vi "rs3 capture single.vi"(0 "queue in":u64, 5 "timeout":u32=5000, 11 "error in (no error)":errorcluster) -> (1 "Capture Error":string="No Error", 3 "RS Format":u16(ring)=6 items=["    RS2_FORMAT_ANY             , /**< When passed to enable stream, librealsense will try to provide best suited format */", "    RS2_FORMAT_Z16             , /**< 16-bit linear depth values. The depth is meters is equal to depth scale * pixel value. */", "    RS2_FORMAT_DISPARITY16     , /**< 16-bit linear disparity values. The depth in meters is equal to depth scale / pixel value. */", "    RS2_FORMAT_XYZ32F          , /**< 32-bit floating point 3D coordinates. */", "    RS2_FORMAT_YUYV            , /**< Standard YUV pixel format as described in https://en.wikipedia.org/wiki/YUV */", "    RS2_FORMAT_RGB8            , /**< 8-bit red, green and blue channels */", "    RS2_FORMAT_BGR8            , /**< 8-bit blue, green, and red channels -- suitable for OpenCV */", "    RS2_FORMAT_RGBA8           , /**< 8-bit red, green and blue channels + constant alpha channel equal to FF */", "    RS2_FORMAT_BGRA8           , /**< 8-bit blue, green, and red channels + constant alpha channel equal to FF */", "    RS2_FORMAT_Y8              , /**< 8-bit per-pixel grayscale image */", "    RS2_FORMAT_Y16             , /**< 16-bit per-pixel grayscale image */", "    RS2_FORMAT_RAW10           , /**< Four 10-bit luminance values encoded into a 5-byte macropixel */", "    RS2_FORMAT_RAW16           , /**< 16-bit raw image */", "    RS2_FORMAT_RAW8            , /**< 8-bit raw image */", "    RS2_FORMAT_UYVY            , /**< Similar to the standard YUYV pixel format, but packed in a different order */", "    RS2_FORMAT_MOTION_RAW      , /**< Raw data from the motion sensor */", "    RS2_FORMAT_MOTION_XYZ32F   , /**< Motion data packed as 3 32-bit float values, for X, Y, and Z axis */", "    RS2_FORMAT_GPIO_RAW        , /**< Raw data from the external sensors hooked to one of the GPIO's */", "    RS2_FORMAT_COUNT             /**< Number of enumeration values. Not a valid input: intended to be used in for-loops. */"], 4 "RS Stream":u16(ring) items=["    RS2_STREAM_ANY,", "    RS2_STREAM_DEPTH                            , /**< Native stream of depth data produced by RealSense device */", "    RS2_STREAM_COLOR                            , /**< Native stream of color data captured by RealSense device */", "    RS2_STREAM_INFRARED                         , /**< Native stream of infrared data captured by RealSense device */", "    RS2_STREAM_FISHEYE                          , /**< Native stream of fish-eye (wide) data captured from the dedicate motion camera */", "    RS2_STREAM_GYRO                             , /**< Native stream of gyroscope motion data produced by RealSense device */", "    RS2_STREAM_ACCEL                            , /**< Native stream of accelerometer motion data produced by RealSense device */", "    RS2_STREAM_GPIO                             , /**< Signals from external device connected through GPIO */", "    RS2_STREAM_COUNT"], 6 "frame out":u64, 8 "width":i32, 10 "Stream type":u16(ring) items=["Depth"=0, "Color (ext.)"=2, "Color (left) "=3, "IR Left"=5, "IR Right"=9, "IR Left (Y16)"=21, "IR Right (Y16)"=25], 12 "index":i32, 14 "height":i32, 15 "error out":errorcluster)   [LabVIEW 2017, in "libRealSense3.lvlib"]
doc: "This VI waits for and returns the FRAME handle of captured data. \nIt also queries the frame profile to identify the type of stream data it was. \nThis type is output into the \"Stream Type\":\n\n0 Depth\n3 Color left\n5 IR Left \n9 IR Right\n21 IR Left (Y16)\n25 IR RIght (Y16)"
uses:
  libRealSense3.lvlib
panel:
  # "RS3 Capture Single"
  # "0   Depth\n3   Color left\n5   IR Left \n9  IR Right\n21  IR Left (Y16)\n25  IR RIght (Y16)"
  # "(C) Intel Corp. 2017,  AGJ"
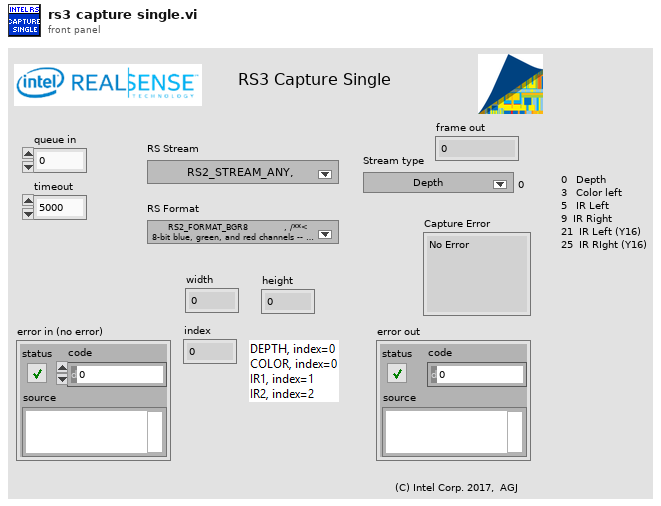
[diagram p1: front panel]
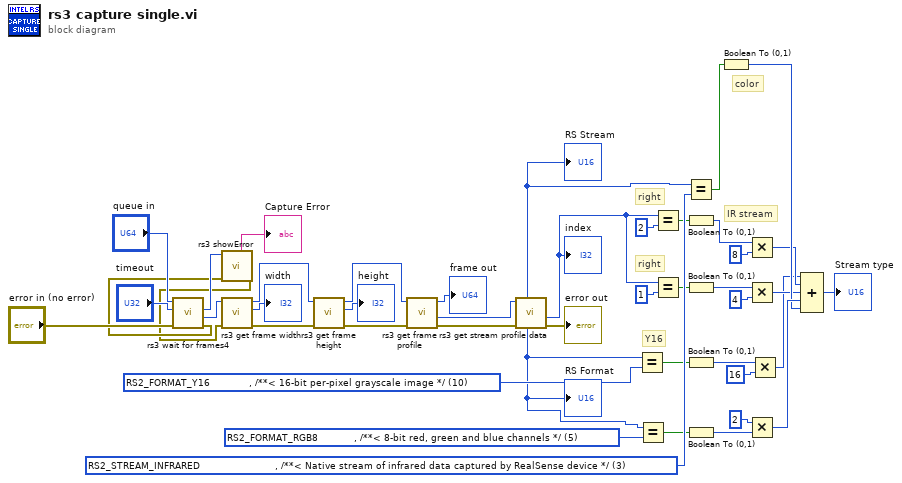
[diagram p0: block diagram]
diagram:
  w7 = u16 10 items=["    RS2_FORMAT_ANY             , /**< When passed to enable stream, librealsense will try to provide best suited format */", "    RS2_FORMAT_Z16             , /**< 16-bit linear depth values. The depth is meters is equal to depth scale * pixel value. */", "    RS2_FORMAT_DISPARITY16     , /**< 16-bit linear disparity values. The depth in meters is equal to depth scale / pixel value. */", "    RS2_FORMAT_XYZ32F          , /**< 32-bit floating point 3D coordinates. */", "    RS2_FORMAT_YUYV            , /**< Standard YUV pixel format as described in https://en.wikipedia.org/wiki/YUV */", "    RS2_FORMAT_RGB8            , /**< 8-bit red, green and blue channels */", "    RS2_FORMAT_BGR8            , /**< 8-bit blue, green, and red channels -- suitable for OpenCV */", "    RS2_FORMAT_RGBA8           , /**< 8-bit red, green and blue channels + constant alpha channel equal to FF */", "    RS2_FORMAT_BGRA8           , /**< 8-bit blue, green, and red channels + constant alpha channel equal to FF */", "    RS2_FORMAT_Y8              , /**< 8-bit per-pixel grayscale image */", "    RS2_FORMAT_Y16             , /**< 16-bit per-pixel grayscale image */", "    RS2_FORMAT_RAW10           , /**< Four 10-bit luminance values encoded into a 5-byte macropixel */", "    RS2_FORMAT_RAW16           , /**< 16-bit raw image */", "    RS2_FORMAT_RAW8            , /**< 8-bit raw image */", "    RS2_FORMAT_UYVY            , /**< Similar to the standard YUYV pixel format, but packed in a different order */", "    RS2_FORMAT_MOTION_RAW      , /**< Raw data from the motion sensor */", "    RS2_FORMAT_MOTION_XYZ32F   , /**< Motion data packed as 3 32-bit float values, for X, Y, and Z axis */", "    RS2_FORMAT_GPIO_RAW        , /**< Raw data from the external sensors hooked to one of the GPIO's */", "    RS2_FORMAT_COUNT             /**< Number of enumeration values. Not a valid input: intended to be used in for-loops. */"] ("RS Format")
  w29 = u16 3 items=["    RS2_STREAM_ANY,", "    RS2_STREAM_DEPTH                            , /**< Native stream of depth data produced by RealSense device */", "    RS2_STREAM_COLOR                            , /**< Native stream of color data captured by RealSense device */", "    RS2_STREAM_INFRARED                         , /**< Native stream of infrared data captured by RealSense device */", "    RS2_STREAM_FISHEYE                          , /**< Native stream of fish-eye (wide) data captured from the dedicate motion camera */", "    RS2_STREAM_GYRO                             , /**< Native stream of gyroscope motion data produced by RealSense device */", "    RS2_STREAM_ACCEL                            , /**< Native stream of accelerometer motion data produced by RealSense device */", "    RS2_STREAM_GPIO                             , /**< Signals from external device connected through GPIO */", "    RS2_STREAM_COUNT"] ("RS Stream")
  w6 = u16 5 items=["    RS2_FORMAT_ANY             , /**< When passed to enable stream, librealsense will try to provide best suited format */", "    RS2_FORMAT_Z16             , /**< 16-bit linear depth values. The depth is meters is equal to depth scale * pixel value. */", "    RS2_FORMAT_DISPARITY16     , /**< 16-bit linear disparity values. The depth in meters is equal to depth scale / pixel value. */", "    RS2_FORMAT_XYZ32F          , /**< 32-bit floating point 3D coordinates. */", "    RS2_FORMAT_YUYV            , /**< Standard YUV pixel format as described in https://en.wikipedia.org/wiki/YUV */", "    RS2_FORMAT_RGB8            , /**< 8-bit red, green and blue channels */", "    RS2_FORMAT_BGR8            , /**< 8-bit blue, green, and red channels -- suitable for OpenCV */", "    RS2_FORMAT_RGBA8           , /**< 8-bit red, green and blue channels + constant alpha channel equal to FF */", "    RS2_FORMAT_BGRA8           , /**< 8-bit blue, green, and red channels + constant alpha channel equal to FF */", "    RS2_FORMAT_Y8              , /**< 8-bit per-pixel grayscale image */", "    RS2_FORMAT_Y16             , /**< 16-bit per-pixel grayscale image */", "    RS2_FORMAT_RAW10           , /**< Four 10-bit luminance values encoded into a 5-byte macropixel */", "    RS2_FORMAT_RAW16           , /**< 16-bit raw image */", "    RS2_FORMAT_RAW8            , /**< 8-bit raw image */", "    RS2_FORMAT_UYVY            , /**< Similar to the standard YUYV pixel format, but packed in a different order */", "    RS2_FORMAT_MOTION_RAW      , /**< Raw data from the motion sensor */", "    RS2_FORMAT_MOTION_XYZ32F   , /**< Motion data packed as 3 32-bit float values, for X, Y, and Z axis */", "    RS2_FORMAT_GPIO_RAW        , /**< Raw data from the external sensors hooked to one of the GPIO's */", "    RS2_FORMAT_COUNT             /**< Number of enumeration values. Not a valid input: intended to be used in for-loops. */"] ("RS Format")
  # "Y16"
  # "right"
  # "IR stream"
  # "color"
  # "right"
  n1 = call "rs3 wait for frames4.vi"("error in (no error)"="error in (no error)", "timeout"="timeout", "Queue in"="queue in") -> (0:"error out"=w2:errorcluster, "frame"=w42:u64, 2:"error out"=w33:u64)  [unwired: 5 in, 1 out]
  n2 = call "rs3 showError.vi"("error in (no error)"=w2, "error"=w33) -> ("error out"=w1:errorcluster, "Error summary"=→"Capture Error":string)  [unwired: 5 in, 3 out]
  n3 = call "rs3 get frame width.vi"("error in (no error)"=w1, "frame in"=w42) -> ("error out"=w36:errorcluster, "width"=→"width":i32, "Frame out"=w40:u64)  [unwired: 6 in, 1 out]
  n4 = call "rs3 get frame height.vi"("error in (no error)"=w36, "frame in"=w40) -> ("error out"=w37:errorcluster, "height"=→"height":i32, "Frame out"=w41:u64)  [unwired: 6 in, 1 out]
  n5 = call "rs3 get frame profile.vi"("error in (no error)"=w37, "Frame"=w41) -> ("error out"=w35:errorcluster, "stream profile"=w34:u64, "frame out"=→"frame out":u64)  [unwired: 6 in, 1 out]
  n6 = call "rs3 get stream profile data.vi"("error in (no error)"=w35, "Profile"=w34) -> ("error out"=→"error out":errorcluster, "index"=w12:i32, "RS Format"=w3:u16, "RS Stream"=w28:u16)  [unwired: 2 in, 4 out]
  "RS Format" <- w3
  "RS Stream" <- w28
  "index" <- w12
  n7 = Equal?(x=w3, y=w7) -> (x = y?=w8:bool)
  n8 = Equal?(x=w3, y=w6) -> (x = y?=w25:bool)
  n9 = Equal?(x=w12, y=2) -> (x = y?=w14:bool)
  n10 = Equal?(x=w12, y=1) -> (x = y?=w26:bool)
  n11 = Equal?(x=w28, y=w29) -> (x = y?=w24:bool)
  n12 = Boolean To (0,1)(Boolean=w14) -> (0, 1=w15:i16)
  n13 = Boolean To (0,1)(Boolean=w26) -> (0, 1=w21:i16)
  n14 = Boolean To (0,1)(Boolean=w8) -> (0, 1=w10:i16)
  n15 = Boolean To (0,1)(Boolean=w25) -> (0, 1=w23:i16)
  n16 = Boolean To (0,1)(Boolean=w24) -> (0, 1=w18:i16)
  n17 = Multiply(x=w15, y=i16 8) -> (x*y=w11:i16)
  n18 = Multiply(x=w21, y=i16 4) -> (x*y=w17:i16)
  n19 = Multiply(x=i16 2, y=w23) -> (x*y=w19:i16)
  n20 = Multiply(x=w10, y=i16 16) -> (x*y=w5:i16)
  n21 = Compound Arithmetic op=ADD(w5, w11, w17, w19, w18) -> (→"Stream type":i16)
